vi "Timer FGV.vi"(7 "Action":T1, 8 "error in (no error)":errorcluster) -> (0 "error out":errorcluster, 3 "Elapsed Time":dbl)   [LabVIEW 2015]
uses:
  Timer Actions.ctl
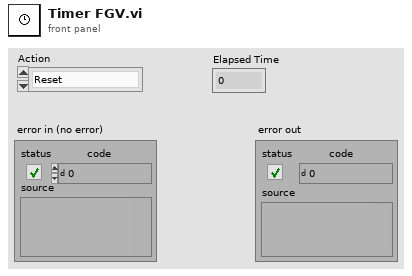
[diagram p1: front panel]
types:
  T1 = typedef "Timer Actions.ctl" = enum16{"Reset", "Get"}
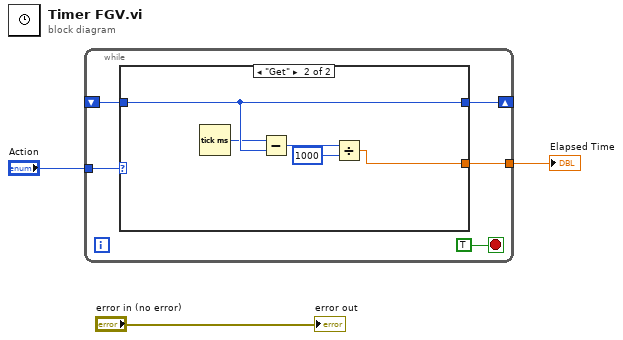
[diagram p0: block diagram]
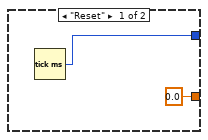
[diagram p2: hidden frame]
diagram:
  n1 = while {
    shift-right: [w6] -> _
    shift-left: _ -> [w5]
    tunnel: "Action" -> [w7]
    tunnel: [w4] -> w1
    stop <- TRUE stop-if-true
    n2 = case shown="\"Get\"" w7 {
      tunnel: [w10 w15] -> w6
      tunnel: w5 -> [_ w15]
      tunnel: [0.0 w11] -> w4
      frame "Reset" {
        n3 = Tick Count (ms)() -> (millisecond timer value=w10:u32)
      }
      frame "Get" {
        n4 = Tick Count (ms)() -> (millisecond timer value=w14:u32)
        n5 = Subtract(x=w14, y=w15) -> (x-y=w13:u32)
        n6 = Divide(x=w13, y=u32 1000) -> (x/y=w11:dbl)
      }
    }
  }
  "Elapsed Time" <- w1
  "error out" <- "error in (no error)"
